vi "Collect Attacks.vi"(6 "Teams in":refnum<class "Team.lvclass">[](array[class]), 9 "New Map in":refnum<class "Map.lvclass">, 11 "Map in":refnum<class "Map.lvclass">) -> (1 "New Map out":refnum<class "Map.lvclass">, 4 "Teams out":refnum<class "Team.lvclass">[](array[class]))   [LabVIEW 2020, in "SquareBattle.lvlib" / "Map.lvclass"]
uses:
  Map.lvclass
  Team/Team.lvclass
  Map.lvclass/Map.ctl
  Position.ctl
  Action.ctl
  Direction Position Offsets.vi
  Normalize Position.vi
  SquareBattle.lvlib
  Square/Square.lvclass
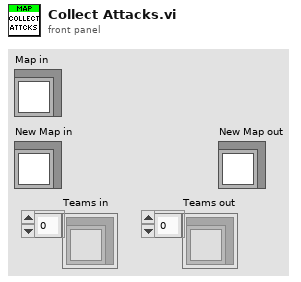
[diagram p1: front panel]
types:
  T1 = typedef "SquareBattle.lvlib/Position.ctl" = cluster{"Row":i32, "Col":i32}
  T2 = typedef "SquareBattle.lvlib/Action.ctl" = enum16{"Wait", "Move", "Attack", "Replicate"}
  T3 = typedef "SquareBattle.lvlib/Run Result.ctl" = cluster{"Action":T2, "Direction":T4, "Replication":refnum<class "Square.lvclass">}
  T4 = typedef "SquareBattle.lvlib/Direction.ctl" = enum16{"NW", "N", "NE", "E", "SE", "S", "SW", "W"}
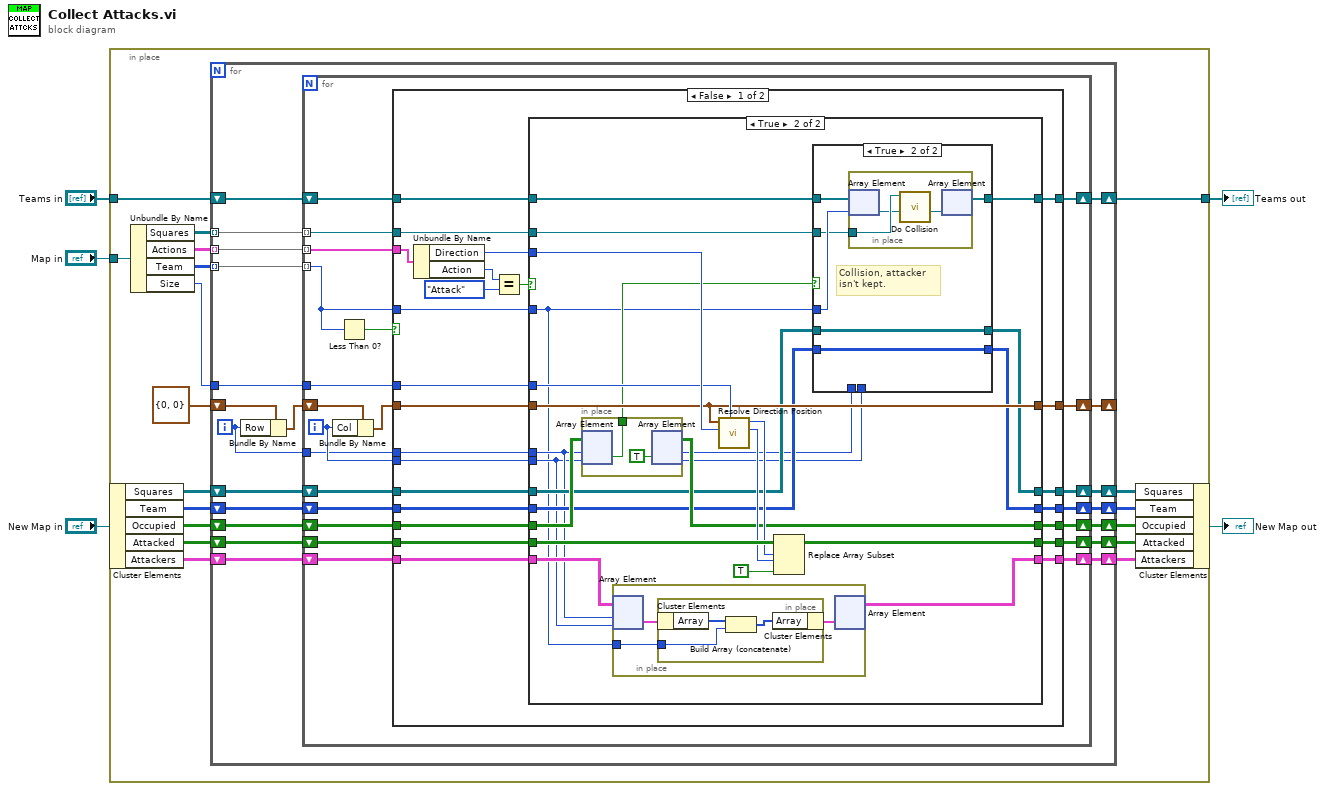
[diagram p0: block diagram]
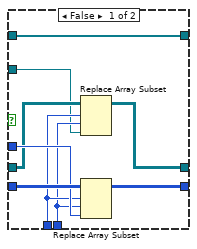
[diagram p3: hidden frame]
diagram:
  n1 = in-place {
    in-place-border: "Map in" -> [w23]
    in-place-border: "Teams in" -> [w9]
    in-place-border: [w8] -> w3
    n2 = in-place-cluster #1("New Map in") -> ("Squares"=w12:refnum<class "Square.lvclass">[][], "Team"=w14:i32[][], "Occupied"=w20:bool[][], "Attacked"=w21:bool[][], "Attackers"=w7:cluster{"Array":i32[]}[][])
    n3 = Unbundle By Name(w23) -> ("Squares"=w16:refnum<class "Square.lvclass">[][], "Actions"=w22:T3[][], "Team"=w17:i32[][], "Size"=w15:i32)
    n4 = for {
      tunnel: w22 -> [w43] mode=indexing
      shift-right: [w40] -> w19
      shift-left: w21 -> [w42]
      shift-right: [w39] -> w18
      shift-left: w20 -> [w41]
      tunnel: w17 -> [w38] mode=indexing
      tunnel: w16 -> [w37] mode=indexing
      tunnel: w15 -> [w36]
      shift-right: [w34] -> w13
      shift-left: w14 -> [w35]
      shift-right: [w32] -> w11
      shift-left: w12 -> [w33]
      shift-right: [w29] -> _
      shift-left: T1 {"Row"=0, "Col"=0} ("Position") -> [w31]
      shift-right: [w26] -> w8
      shift-left: w9 -> [w27]
      shift-right: [w24] -> w6
      shift-left: w7 -> [w25]
      i -> [w28]
      n5 = Bundle By Name(cluster=w31, "Row"=w28) -> (w30:T1)
      n6 = for {
        tunnel: w43 -> [w63] mode=indexing
        shift-right: [w58] -> w40
        shift-left: w42 -> [w59]
        shift-right: [w57] -> w39
        shift-left: w41 -> [w60]
        tunnel: w38 -> [w64] mode=indexing
        tunnel: w37 -> [w62] mode=indexing
        tunnel: w36 -> [w61]
        shift-right: [w55] -> w34
        shift-left: w35 -> [w56]
        shift-right: [w53] -> w32
        shift-left: w33 -> [w54]
        shift-right: [w50] -> w29
        shift-left: w30 -> [w52]
        tunnel: w28 -> [w48]
        shift-right: [w46] -> w26
        shift-left: w27 -> [w47]
        shift-right: [w44] -> w24
        shift-left: w25 -> [w45]
        i -> [w49]
        n7 = Bundle By Name(cluster=w52, "Col"=w49) -> (w51:T1)
        n8 = Less Than 0?(x=w64) -> (x < 0?=w65:bool)
        n9 = case shown="False" w65 {
          tunnel: w64 -> [w69 _]
          tunnel: w63 -> [w89 _]
          tunnel: w62 -> [w80 _]
          tunnel: w61 -> [w73 _]
          tunnel: w60 -> [w84 w153]
          tunnel: w59 -> [w83 w154]
          tunnel: [w74 w154] -> w58
          tunnel: [w75 w153] -> w57
          tunnel: w56 -> [w85 w152]
          tunnel: [w76 w152] -> w55
          tunnel: w54 -> [w86 w151]
          tunnel: [w77 w151] -> w53
          tunnel: w51 -> [w78 w150]
          tunnel: [w79 w150] -> w50
          tunnel: w49 -> [w72 _]
          tunnel: w48 -> [w71 _]
          tunnel: w47 -> [w70 w149]
          tunnel: [w68 w149] -> w46
          tunnel: w45 -> [w67 w148]
          tunnel: [w66 w148] -> w44
          frame False {
            n10 = Unbundle By Name(w89) -> ("Direction"=w81:T4, "Action"=w88:T2)
            n11 = Equal?(x=w88, y=Action."Attack") -> (x = y?=w82:bool)
            n12 = case shown="True" w82 {
              tunnel: w86 -> [w95 w107]
              tunnel: w85 -> [w94 w106]
              tunnel: w84 -> [w93 w113]
              tunnel: w83 -> [w92 w119]
              tunnel: w81 -> [_ w121]
              tunnel: w80 -> [_ w109]
              tunnel: [w96 w114] -> w79
              tunnel: w78 -> [w96 w114]
              tunnel: [w95 w105] -> w77
              tunnel: [w94 w104] -> w76
              tunnel: [w93 w112] -> w75
              tunnel: [w92 w115] -> w74
              tunnel: w73 -> [_ w120]
              tunnel: w72 -> [_ w99]
              tunnel: w71 -> [_ w100]
              tunnel: w70 -> [w91 w110]
              tunnel: w69 -> [_ w98]
              tunnel: [w91 w108] -> w68
              tunnel: w67 -> [w90 w101]
              tunnel: [w90 w97] -> w66
              frame False {
              }
              frame True {
                n13 = in-place {
                  in-place-border: [w147] -> w111
                  n14 = in-place-array #2(w113, w100, w99) -> (w147:bool)
                  n15 = in-place-array #2(TRUE ("element")) -> (w112:bool[][], w103:i32, w102:i32)
                }
                n16 = in-place {
                  in-place-border: w98 -> [w122]
                  n17 = in-place-array #3(w101, w100, w99) -> (w124:cluster{"Array":i32[]})
                  n18 = in-place {
                    in-place-border: w122 -> [w126]
                    n19 = in-place-cluster #4(w124) -> ("Array"=w127:i32[])
                    n20 = Build Array (concatenate)(w127, w126) -> (w125:i32[])
                    n21 = in-place-cluster #4("Array"=w125) -> (w123:cluster{"Array":i32[]})
                  }
                  n22 = in-place-array #3(w123) -> (w97:cluster{"Array":i32[]}[][])  [unwired: 2 out]
                }
                n23 = call "Resolve Direction Position.vi"("Board Size"=w120, "Direction"=w121, "From"=w114) -> ("Col"=w118:i32, "Row"=w117:i32)  [unwired: 6 in, 1 out]
                n24 = Replace Array Subset(array=w119, new element=TRUE ("new element/subarray"), index (row)=w117, index (col)=w118) -> (w115:bool[][])
                n25 = case shown="True" w111 {
                  tunnel: w110 -> [w129 w142]
                  tunnel: w109 -> [w128 w140]
                  tunnel: w98 -> [w134 w141]
                  tunnel: [w129 w139] -> w108
                  tunnel: w107 -> [w133 w138]
                  tunnel: w106 -> [w136 w137]
                  tunnel: [w130 w138] -> w105
                  tunnel: [w135 w137] -> w104
                  tunnel: w103 -> [w132 _]
                  tunnel: w102 -> [w131 _]
                  frame False {
                    n26 = Replace Array Subset(array=w133, new element=w128, index (row)=w132, index (col)=w131) -> (w130:refnum<class "Square.lvclass">[][])
                    n27 = Replace Array Subset(array=w136, new element=w134, index (row)=w132, index (col)=w131) -> (w135:i32[][])
                  }
                  frame True {
                    # "Collision, attacker isn't kept."
                    n28 = in-place {
                      in-place-border: w140 -> [w145]
                      n29 = in-place-array #5(w142, w141) -> (w144:refnum<class "Team.lvclass">)
                      n30 = call "Do Collision.vi"("Team in"=w144, "Square"=w145) -> ("Team out"=w143:refnum<class "Team.lvclass">)  [unwired: 9 in]
                      n31 = in-place-array #5(w143) -> (w139:refnum<class "Team.lvclass">[])  [unwired: 1 out]
                    }
                  }
                }
              }
            }
          }
          frame True {
            # "Empty position, ain't gotta do anything."
          }
        }
      }
    }
    n32 = in-place-cluster #1("Squares"=w11, "Team"=w13, "Occupied"=w18, "Attacked"=w19, "Attackers"=w6) -> (→"New Map out":refnum<class "Map.lvclass">)
  }
  "Teams out" <- w3
